vi "RT Inhibit Bus A - Dual RT.vi"(8 "error in (no error)":errorcluster, 11 "1553 Unit Test in":refnum<class "Remote Terminal.lvclass">) -> (0 "error out":errorcluster, 3 "1553 Unit Test out":refnum<class "Remote Terminal.lvclass">)   [LabVIEW 2020, in "Unit Tests.lvlib" / "Remote Terminal.lvclass"]
uses:
  Remote Terminal.lvclass
  Remote Terminal/TypeDefs/RT Configuration.ctl
  Remote Terminal/TypeDefs/RT-RT Timeout.ctl
  Remote Terminal/TypeDefs/Mode Code 17 Sync Configuration.ctl
  Remote Terminal/TypeDefs/RT Timetag Configuration.ctl
  Remote Terminal/TypeDefs/RT Command Config.ctl
  Frames & Messages/TypeDefs/Command Type.ctl
  Frames & Messages/TypeDefs/Command SubAddress.ctl
  Frames & Messages/TypeDefs/Command Word Count.ctl
  Frames & Messages/TypeDefs/Simplified Parameter Data Table.ctl
  Frames & Messages/TypeDefs/Scaling Information.ctl
  Remote Terminal.lvclass/Remote Terminal.ctl
  Remote Terminal/Remote Terminal.lvclass
  C:/Users/MattJ/Desktop/git/bci-1553-labview-api/src/1553 SubComponent/1553 SubComponent.lvclass
  <vilib>/addons/_JKI Toolkits/Caraya/classes/Assert/Assert True.vi
  1553 Session/1553 Session.lvclass
  Dependencies/FPGA Interface/FPGA Interface.lvclass
  BCI-1553 API.lvlib
  1553 Component/1553 Component.lvclass
  <vilib>/addons/_JKI Toolkits/Caraya/classes/Test/Test.lvclass
  <vilib>/addons/_JKI Toolkits/Caraya/classes/Assert/Assert.lvclass
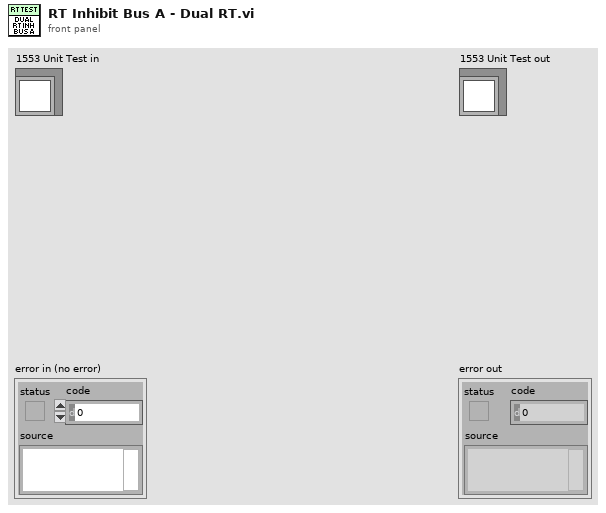
[diagram p1: front panel]
types:
  T1 = typedef "BCI-1553 API.lvlib/Remote Terminal.lvclass/RT Configuration.ctl" = cluster{"RT-RT Timeout":T2, "Inhibit Bus A":bool, "Inhibit Bus B":bool, "Broadcast CMD Invalid":bool, "UnDef MCs Invalid":bool, "Notice 2 Data Storage":bool, "SMCP":bool, "Temp RX Buffer":bool, "Alt BIT Enable":bool, "Auto Bus Shutdown":bool, "MC 16 SR Reset":bool, "MC 17 Sync":T3, "MC 8 Reset":bool, "Remote Terminal Timetag Config":T4}
  T2 = typedef "BCI-1553 API.lvlib/Remote Terminal.lvclass/RT-RT Timeout.ctl" = enum16{"57us", "62us", "100us", "180us"}
  T3 = typedef "BCI-1553 API.lvlib/Remote Terminal.lvclass/Mode Code 17 Sync Configuration.ctl" = enum16{"Sync if Bit 0 = 1", "Sync if Bit 0 = 0", "Sync Unconditionally"}
  T4 = typedef "BCI-1553 API.lvlib/Remote Terminal.lvclass/RT Timetag Configuration.ctl" = enum16{"Disabled", "2us", "4us", "8us", "16us", "32us", "64us"}
  T5 = typedef "BCI-1553 API.lvlib/Remote Terminal.lvclass/RT Command Config.ctl" = cluster{"Command Type":T6, "SubAddress":T7, "Word Count\\Mode Code":T8, "Initial Data":u16[], "Data Fields":T9[]}
  T6 = typedef "BCI-1553 API.lvlib/Command Type.ctl" = enum16{"Transmit", "Receive"}
  T7 = typedef "BCI-1553 API.lvlib/Command SubAddress.ctl" = enum16{"Mode Code", "1", "2", "3", "4", "5", "6", "7", "8", "9", "10", "11", "12", "13", "14", "15", "16", "17", "18", "19", "20", "21", "22", "23", "24", "25", "26", "27", "28", "29", "30"}
  T8 = typedef "BCI-1553 API.lvlib/Command Word Count.ctl" = enum16{"1", "2", "3", "4", "5", "6", "7", "8", "9", "10", "11", "12", "13", "14", "15", "16", "17", "18", "19", "20", "21", "22", "23", "24", "25", "26", "27", "28", "29", "30", "31", "32"}
  T9 = typedef "BCI-1553 API.lvlib/Simplified Parameter Data Table.ctl" = cluster{"Parameter Name":string, "Base Word":u16, "Scaling Info":T10}
  T10 = typedef "BCI-1553 API.lvlib/Scaling Information.ctl" = cluster{"Bit Offset":i32, "Bit Count":i32, "LSB Resolution":dbl, "2's Complement":bool, "Big Endian":bool, "Sign Bit":bool}
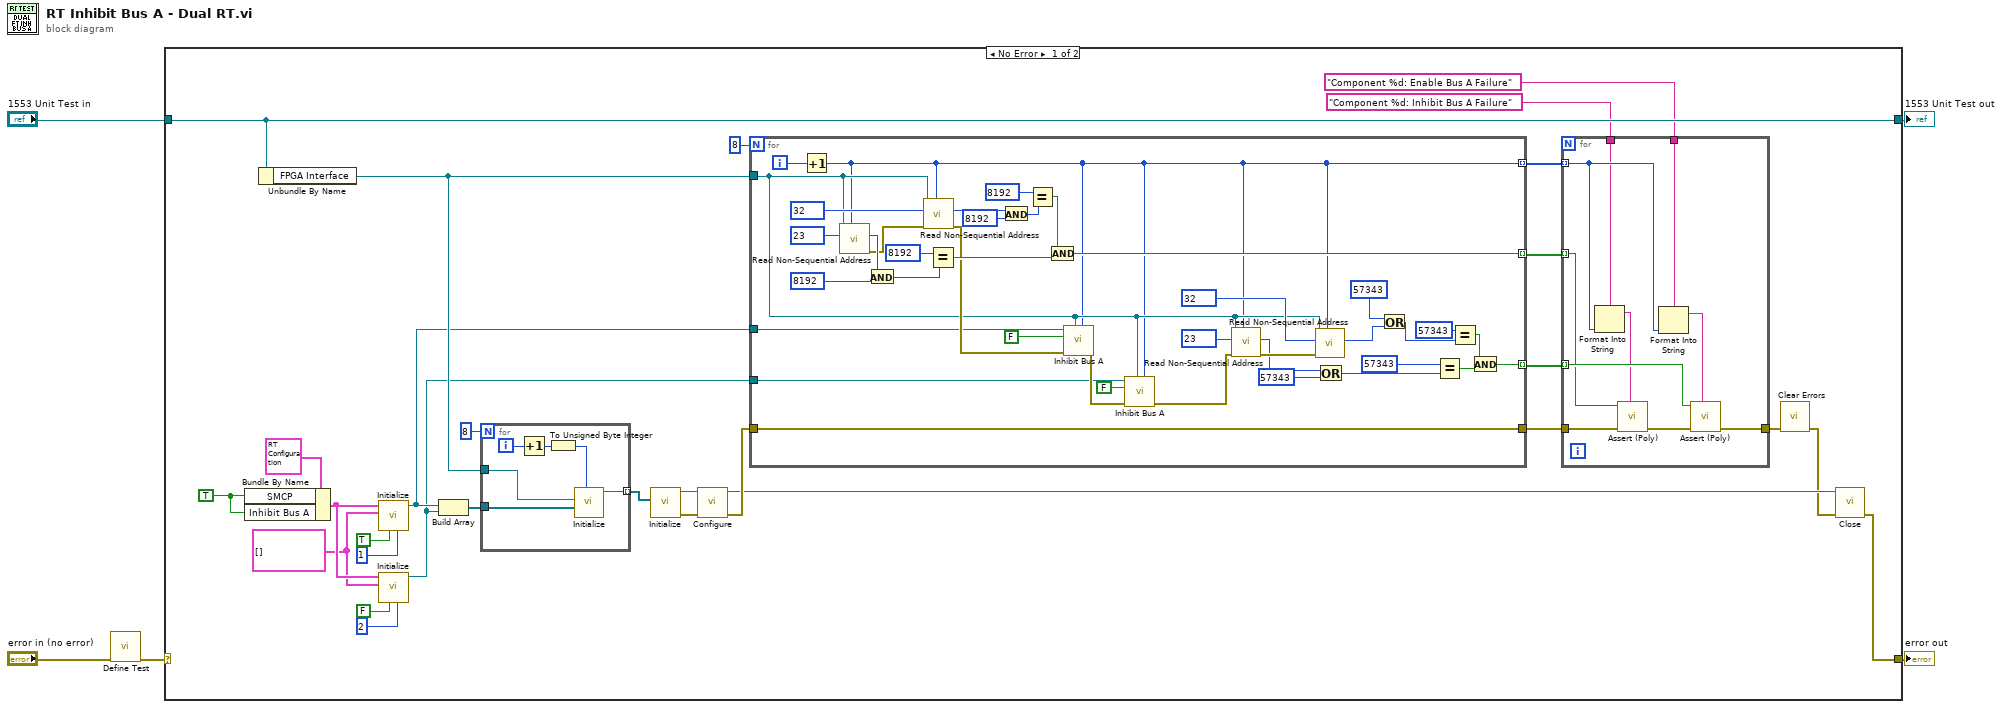
[diagram p0: block diagram]
diagram:
  n1 = call <vilib>:"Define Test.vi"("error in (no error)"="error in (no error)") -> ("error out"=w1:errorcluster)  [unwired: 9 in, 1 out]
  n2 = case shown="No Error" w1 {
    selector: w1 -> [_ w91]
    tunnel: [w6 w91] -> w5
    tunnel: [w24 w90] -> w3
    tunnel: "1553 Unit Test in" -> [w24 w90]
    frame No Error {
      w27 = T5[] [] ("RT Commands")
      w31 = TRUE ("SMCP")
      n3 = Bundle By Name(cluster=T1 {"RT-RT Timeout"=enum."57us", "Inhibit Bus A"=FALSE, "Inhibit Bus B"=FALSE, "Broadcast CMD Invalid"=FALSE, "UnDef MCs Invalid"=FALSE, "Notice 2 Data Storage"=FALSE, "SMCP"=FALSE, "Temp RX Buffer"=FALSE, "Alt BIT Enable"=FALSE, "Auto Bus Shutdown"=FALSE, "MC 16 SR Reset"=FALSE, "MC 17 Sync"=enum."Sync if Bit 0 = 1", "MC 8 Reset"=FALSE, "Remote Terminal Timetag Config"=enum."Disabled"} ("RT Configuration"), "SMCP"=w31, "Inhibit Bus A"=w31) -> (w28:T1)
      n4 = Unbundle By Name(w24) -> ("FPGA Interface"=w18:refnum<class "FPGA Interface.lvclass">)
      n5 = call "Initialize.vi"("Terminal Address"=u8 1 ("RT Address (0-30)"), "RT 1?"=TRUE, "RT Commands"=w27, "RT Configuration"=w28) -> ("Remote Terminal out"=w17:refnum<class "Remote Terminal.lvclass">)  [unwired: 6 in, 1 out]
      n6 = call "Initialize.vi"("Terminal Address"=u8 2 ("RT Address (0-30)"), "RT 1?"=FALSE, "RT Commands"=w27, "RT Configuration"=w28) -> ("Remote Terminal out"=w16:refnum<class "Remote Terminal.lvclass">)  [unwired: 6 in, 1 out]
      n7 = Build Array(w17, w16) -> (w25:refnum<class "Remote Terminal.lvclass">[])
      n8 = for {
        N: 8 -> [_]
        tunnel: [w87] -> w23 mode=indexing
        tunnel: w25 -> [w86]
        tunnel: w18 -> [w85]
        i -> [w89]
        n9 = Increment(x=w89) -> (x+1=w84:i32)
        n10 = To Unsigned Byte Integer(number=w84) -> (unsigned 8bit integer=w88:u8)
        n11 = call "Initialize.vi"("Component ID (1-8)"=w88, "SubComponents"=w86, "FPGA Interface"=w85) -> ("1553 Component out"=w87:refnum<class "1553 Component.lvclass">)  [unwired: 7 in, 1 out]
      }
      n12 = call "Initialize.vi"("Components"=w23) -> ("error out"=w21:errorcluster, "1553 Board out"=w22:refnum<class "1553 Session.lvclass">)  [unwired: 9 in]
      n13 = call-dynamic "Configure.vi"("error in (no error)"=w21, "1553 Board in"=w22) -> ("error out"=w19:errorcluster, "1553 Board out"=w8:refnum<class "1553 Session.lvclass">)  [unwired: 8 in]
      n14 = for {
        N: 8 -> [_]
        tunnel: w19 -> [w78]
        tunnel: [w78] -> w12
        tunnel: w18 -> [w59]
        tunnel: [w72] -> w15 mode=indexing
        tunnel: [w51] -> w13 mode=indexing
        tunnel: w17 -> [w54]
        tunnel: w16 -> [w53]
        tunnel: [w52] -> w14 mode=indexing
        i -> [w79]
        n15 = Increment(x=w79) -> (x+1=w51:i32)
        n16 = call-dynamic "Read Non-Sequential Address.vi"("Target IC (1-8)"=w51, "Address"=u16 23, "FPGA Interface in"=w59) -> ("error out"=w68:errorcluster, "Data"=w80:u16)  [unwired: 7 in]
        n17 = And(x=w80, y=u16 8192) -> (x .and. y?=w71:u16)
        n18 = call-dynamic "Read Non-Sequential Address.vi"("Target IC (1-8)"=w51, "error in (no error)"=w68, "Address"=u16 32, "FPGA Interface in"=w59) -> ("error out"=w60:errorcluster, "Data"=w69:u16)  [unwired: 6 in]
        n19 = Equal?(x=u16 8192, y=w71) -> (x = y?=w73:bool)
        n20 = And(x=w69, y=u16 8192) -> (x .and. y?=w70:u16)
        n21 = Equal?(x=u16 8192, y=w70) -> (x = y?=w74:bool)
        n22 = And(x=w74, y=w73) -> (x .and. y?=w72:bool)
        n23 = call-dynamic "Inhibit Bus A.vi"("Component ID"=w51, "FPGA Interface"=w59, "error in (no error)"=w60, "Inhibit Bus A?"=FALSE ("Bus B Inhibited?"), "Remote Terminal in"=w54) -> ("error out"=w58:errorcluster)  [unwired: 5 in, 1 out]
        n24 = call-dynamic "Inhibit Bus A.vi"("Component ID"=w51, "FPGA Interface"=w59, "error in (no error)"=w58, "Inhibit Bus A?"=FALSE ("Bus B Inhibited?"), "Remote Terminal in"=w53) -> ("error out"=w55:errorcluster)  [unwired: 5 in, 1 out]
        n25 = call-dynamic "Read Non-Sequential Address.vi"("Target IC (1-8)"=w51, "error in (no error)"=w55, "Address"=u16 23, "FPGA Interface in"=w59) -> ("error out"=w61:errorcluster, "Data"=w49:u16)  [unwired: 6 in]
        n26 = call-dynamic "Read Non-Sequential Address.vi"("Target IC (1-8)"=w51, "error in (no error)"=w61, "Address"=u16 32, "FPGA Interface in"=w59) -> ("Data"=w47:u16)  [unwired: 6 in, 1 out]
        n27 = Or(x=w49, y=u16 57343) -> (x .or. y?=w48:u16)
        n28 = Or(x=u16 57343, y=w47) -> (x .or. y?=w46:u16)
        n29 = Equal?(x=u16 57343, y=w48) -> (x = y?=w62:bool)
        n30 = Equal?(x=u16 57343, y=w46) -> (x = y?=w63:bool)
        n31 = And(x=w63, y=w62) -> (x .and. y?=w52:bool)
      }
      n32 = for {
        tunnel: w15 -> [w41] mode=indexing
        tunnel: w14 -> [w42] mode=indexing
        tunnel: w13 -> [w38] mode=indexing
        tunnel: w12 -> [w44]
        tunnel: "Component %d: Inhibit Bus A Failure" ("custom report message (\"\")") -> [w37]
        tunnel: "Component %d: Enable Bus A Failure" ("custom report message (\"\")") -> [w36]
        tunnel: [w35] -> w9
        n33 = Format Into String(format string=w37, w38) -> (resulting string=w40:string)  [unwired: 2 in, 1 out]
        n34 = call-poly <vilib>:"Assert (Poly).vi"("Label"=w40, "error in (no error)"=w44, "True?"=w41) -> ("error out"=w43:errorcluster)  [unwired: 7 in, 1 out]
        n35 = Format Into String(format string=w36, w38) -> (resulting string=w39:string)  [unwired: 2 in, 1 out]
        n36 = call-poly <vilib>:"Assert (Poly).vi"("Label"=w39, "error in (no error)"=w43, "True?"=w42) -> ("error out"=w35:errorcluster)  [unwired: 7 in, 1 out]
      }
      n37 = call <vilib>:"Clear Errors.vi"("error in (no error)"=w9) -> ("error out"=w7:errorcluster)  [unwired: 5 in, 1 out]
      n38 = call-dynamic "Close.vi"("error in (no error)"=w7, "1553 Board in"=w8) -> ("error out"=w6:errorcluster)  [unwired: 9 in]
    }
    frame Error {
    }
  }
  "error out" <- w5
  "1553 Unit Test out" <- w3
